vi "WB_print_sub.vi"(1 "최소값":dbl=-2.4903133, 2 "최대값":dbl=1.9686242, 3 "배열":dbl[][](array[numeric])) -> (0 "?":dbl[][](graph)=[[0.019402362, -0.056784116, 0.07198692, 0.023335427, 0.01416415, 0.050220422, -0.07103005, 0.081241615, -0.073664345, -0.05044797, -0.05076698, 0.06311553, 0.061175354, 0.052017786, -0.048248764, -0.08574579, 0.03520029, 0.001996823, 0.04126946, -0.043121457, 0.084707774, -0.06773842, 0.070435666, 0.019763917, -0.059031256, -0.03149846, -0.08095915, 0.004533172], [0.028954692, -0.025707066, -0.05200914, -0.003957868, 0.023727901, -0.06592558, -0.02315136, -0.2734161, -0.20163584, -0.36126682, -0.3774755, -0.14096943, -0.2054312, -0.3512236, 0.33971533, 0.25994176, -0.46906397, -0.70744854, -0.19329818, -0.088722445, 0.036387537, 0.0862372, 0.016047418, 0.06599588, 0.012692414, -0.077935, 0.05922284, 0.05609662], [0.013729125, 0.08213016, 0.06034646, -0.05076416, 0.06025117, -0.15579464, -0.16772258, -0.3223184, -0.37558174, -0.3752564, -0.67335427, -0.49895945, -0.08313592, 0.2052238, 0.2807211, 0.57371145, 0.41389152, -0.17161524, -0.61246336, -0.5017266, -0.50128746, -0.53516656, -0.27541342, -0.3253776, -0.19609226, -0.11948956, -0.012640931, -0.0647767], [-0.015670069, -0.06668488, 0.28268385, 0.20505649, -0.23857276, -0.39677197, -0.38728097, -0.40845335, -0.7503476, -0.4884504, -0.6518539, -0.7594363, -0.24838643, -0.16143909, -0.45154887, -0.02543016, 0.003746802, -0.37966758, -0.49458778, -0.44614837, -0.5836974, -0.41483384, -0.53961504, -0.81955177, -0.83781636, -0.50216895, -0.26348847, -0.076926686], [0.05106411, -0.07743591, 0.26234427, 0.2574695, 0.16226213, -0.46701786, -0.42931813, -0.2339498, -0.14295034, -0.2446104, 0.02086417, -0.32185107, -0.104272395, 0.15050568, 0.027467467, 0.03022217, -0.108522505, -0.27108124, -0.11329941, 0.026872164, 0.048474103, -0.027454505, -0.25504008, -0.26145422, -0.76783425, -0.92602754, -0.58093053, -0.37015644], [0.076194845, -0.034185234, 0.40671673, 0.37028506, 0.41466984, -0.31411722, -0.61910045, -0.59914446, -0.7287402, -0.5391061, -0.2669772, -0.44680798, -0.33798522, -0.1343784, -0.07999179, 0.089457855, -0.19059445, -0.3474572, -0.2032107, -0.083512895, -0.0830359, 0.221656, 0.19037572, 0.12669519, -0.074350126, -1.1324757, -0.4394831, -0.30350068], [-0.032071892, 0.05306862, -0.2989132, 0.21729691, 0.3500755, -0.73872447, -0.8738451, -0.9976445, -0.5223479, -0.3658319, -0.2307682, -0.034148972, -0.13845769, -0.18013148, -0.2361024, -0.31985897, -0.43676993, -0.34739915, -0.06262585, -0.18276054, 0.06466541, 0.08421242, 0.07748312, 0.11180859, -0.21580644, -1.4230266, -0.44195205, -0.3313512], [0.038363524, -0.30228248, -0.21182631, -0.057430062, -0.16909048, -0.92691547, -1.1927773, -0.59489316, -0.5452894, -0.23881502, -0.037728827, -0.038009986, 0.02855738, -0.09971486, -0.14617823, -0.3563637, -0.3384605, -0.24687314, -0.11111135, 0.07221237, 0.033493813, -0.005995454, -0.036368825, -0.15205514, -0.9522951, -1.3690672, -0.43376705, -0.36297065], [0.04789371, -0.27008292, -0.36039582, 0.21856155, -0.37664315, -1.0078262, -0.7442325, -0.44629014, -0.74698794, -0.41905984, -0.084661156, -0.21115676, -0.017576342, 0.072085276, 0.10647539, -0.055365387, -0.1613902, 0.027296007, -0.10239959, -0.034265842, -0.1916164, -0.20936437, -0.24815829, -0.66299695, -1.2413676, -1.1379274, -0.4866338, -0.21672283], [-0.03621333, -0.32016924, -0.35166052, -0.19059004, -0.7421054, -0.6603438, -0.2594525, -0.28854498, -0.54254127, -0.586046, -0.18177606, -0.035845097, -0.14068633, 0.021429166, 0.24718617, 0.54646474, 0.2706092, -0.023800315, -0.11697391, -0.32499748, -0.3964098, -0.17136137, -0.378053, -0.8393874, -1.0225842, -1.1827171, -0.2501431, -0.12847507], [0.045761995, 0.080762595, -0.27182245, -0.26441163, -0.6160039, -0.8418736, -0.5958423, -0.41623044, -0.29561433, -0.5286718, -0.13444705, -0.048691455, -0.06864151, 0.1826969, 0.6635885, 0.802045, 0.32688302, 0.0874516, -0.17387727, -0.2563993, -0.30054188, -0.096157655, -0.508509, -0.99769956, -1.4066856, -0.29529485, -0.37173674, 0.21905021], [-0.07151403, 0.28909746, 0.38781136, -0.26616985, -0.4273282, -0.41229233, -0.8697481, -0.5518835, -0.31008196, -0.2774829, -0.26617262, -0.15640731, -0.10818419, 0.24041, 0.79541355, 0.70669216, 0.28055012, -0.16330147, -0.10160323, -0.2256082, -0.35910672, -0.39827135, -0.650711, -0.62799734, -0.90181077, -0.107671015, -0.36124784, 0.22384478], [0.078392126, 0.031860493, -0.25298005, 0.095670424, -0.14538823, -0.16609928, -0.31244653, -0.12862818, -0.22139308, 0.07183458, -0.32371405, -0.4855172, -0.08327049, 0.3265337, 0.78024745, 0.60129076, 0.18782617, -0.01853502, -0.07388906, -0.40313932, -0.40507895, -0.009898128, -0.27054566, -0.34444198, -0.7273675, -0.2863849, -0.42149025, 0.041592613], [0.21364997, -0.007809334, -0.15489164, 0.41396883, 0.031446937, -0.14940584, -0.2472778, -0.22871476, 0.32454446, -0.028100867, -0.65081227, -0.552141, -0.016222754, 0.30621958, 0.6353163, 0.6064552, 0.1867488, 0.19777592, -0.1788572, -0.6515122, -0.52407956, -0.11200111, -0.4531192, -0.592242, -0.7931037, -0.4800189, -0.43356013, -0.09559373], [0.041847475, 0.020147942, 0.28636876, 0.3035632, 0.3176007, -0.2528747, -0.78754634, -0.18334779, 0.092457, -0.2796707, -0.74587876, -0.5658111, 0.000195621, 0.30102542, 0.6712702, 0.49273783, 0.22195052, -0.16626519, -0.41114998, -0.5848261, -0.4108646, -0.18204437, -0.21483289, -0.14545862, 0.025073398, -0.07972018, 0.14786825, 0.0397756], [0.007859804, 0.004111923, 0.3043381, 0.38932654, 0.4320326, -0.4698006, -0.9373428, -0.04405305, -0.023937216, -0.47727737, -0.483351, -0.083477095, 0.21139918, 0.5714958, 0.8108114, 0.20742717, 0.18971094, -0.5720092, -0.8250202, -1.2184142, -1.1274087, -0.2133971, -0.31071362, -0.5049326, -0.18142083, -0.24756274, 0.030007659, -0.2307325], [0.034503534, 0.30741704, 0.3961975, -0.028361622, 0.16783519, -0.7315894, -0.8071333, -0.37223402, -0.27927428, 0.0536947, -0.21464181, -0.053445697, -0.011839257, 0.4265288, 0.6584135, 0.006877806, -0.117410704, -0.88479674, -0.9323623, -1.306204, -0.35932663, -0.20176698, -0.26285505, -0.79386646, -0.49305102, -0.92046, -0.20253757, -0.4379618], [0.0269147, 0.26754153, 0.17135796, -0.20873298, 0.11994213, -0.8284057, -0.88438743, -0.502535, -0.112462565, -0.18551545, -0.047672696, -0.33874467, 0.074904464, 0.40984982, 0.6418728, -0.05189987, -0.48060784, -0.8236671, -0.42577484, -0.22257994, -0.042787, -0.009383095, 0.05736418, -0.19098903, -0.4478566, -1.0353278, -0.020705368, -0.39874083], [0.1397072, 0.45009655, -0.064224996, -0.3019297, -0.8661276, -1.3250548, -1.2598255, -0.5243417, -0.058559388, -0.09852703, -0.3158096, -0.19829708, -0.0714448, 0.22167754, 0.2854061, -0.3002683, -0.59488386, -0.2821777, 0.028929045, 0.05826009, 0.33111486, 0.16548227, -0.21062346, -0.25565898, -0.5472606, -0.28622505, 0.18191522, 0.41757488], [0.23692198, 0.29008064, 0.082759045, -0.002741147, -0.8795839, -1.4149228, -0.5514523, -0.000486821, -0.03483119, 0.06705211, -0.12580939, -0.05553379, 0.0186108, 0.24032596, 0.005597983, -0.06941267, 0.16518432, -0.06645737, 0.19766212, 0.38022786, 0.09240109, -0.013227117, -0.25650293, -0.044998907, 0.12227106, 0.17152156, 0.18103345, 0.41024154], [-0.06607313, -0.020586662, -0.3017442, -0.48487973, -0.623512, -0.7337084, -0.13421166, -0.012992498, 0.19180049, 0.10447126, 0.17092228, 0.22486123, 0.0976739, -0.06349748, 0.106518574, 0.05040216, 0.36003187, 0.276737, 0.49036795, 0.30218476, 0.11204288, 0.12559855, -0.35291293, -0.35144538, 0.014885792, 0.005825452, 0.29019934, 0.21266916], [0.27878812, 0.15665133, -0.003313494, 0.12400361, 0.2629784, 0.37134543, 0.2215543, 0.11155561, 0.15902479, 0.20833528, 0.32967663, 0.037060052, -0.08899602, -0.16459641, 0.1264346, 0.2089554, 0.1434192, 0.06803246, 0.4307756, 0.24303465, 0.18769139, 0.25835752, -0.4969824, -0.73953736, -0.10242521, -0.112113826, 0.003337876, -0.0351161], [0.28544542, 0.1967097, -0.006959932, -0.20673351, 0.026372466, 0.94482493, 0.4533628, 0.026862903, 0.17517203, 0.20571615, -0.039798018, -0.29742217, -0.3459068, -0.36140463, 0.0369192, -0.012902046, 0.048173387, 0.33128628, 0.47379583, 0.3349553, 0.25610295, -0.08089572, -0.5139698, -0.07225746, -0.5919201, 0.19126964, 0.36402228, 0.075980864], [-0.04799637, 0.022139437, -0.08066415, -0.45350027, -0.36171135, 0.48501188, 0.40540573, 0.07247676, -0.002596119, -0.068791166, -0.120647185, -0.13058528, 0.06652875, -0.15032628, -0.2481706, 0.10068886, 0.17316899, 0.44682083, 0.07280411, 0.03211489, -0.29994527, -0.5088104, -0.42009258, -0.87431175, -0.06847369, 0.17766212, 0.52052814, 0.008205421], [-0.08633989, 0.050158076, -0.10934232, -0.43204042, -0.7932491, -0.085638694, -0.04620965, -0.21960713, -0.3608294, -0.15517698, -0.31756258, -0.34403557, -0.22502212, -0.47006503, -0.24211344, -0.36654466, -0.69102883, -0.022553908, -0.07223295, 0.08607136, -0.40333796, -0.29468244, -0.44569877, -0.06304068, -0.17344941, 0.35010365, 0.27814704, 0.006576605], [-0.05087135, -0.08338762, -0.030791346, -0.4005939, -0.85698, -0.90138805, -0.79291576, -0.93168545, -0.4134845, -0.50070626, -1.4878545, -1.4652365, -0.84761375, -0.87468684, -0.76639235, -1.0541568, -1.6761183, -1.4510397, -1.2478479, -1.2098646, -0.7164307, -0.44639748, -0.21093823, -0.2979916, -0.3668138, 0.048997097, -0.07975093, -0.07314849], [0.064261444, -0.012364283, 0.051179014, -0.1375661, -0.27762103, -0.35109448, -0.44071844, -0.44467148, -0.74206126, -0.91204447, -0.8158255, -0.9406752, -1.1595905, -0.9655593, -1.0871019, -0.8791337, -0.9534564, -0.90534633, -0.59114176, -0.49164557, -0.23583324, -0.3829994, -0.38570908, -0.29194045, -0.00429406, -0.012259826, 0.02296777, -0.039393578], [-0.041495476, -0.061708644, 0.040426068, -0.068808526, -0.008004427, -0.0743755, -0.03914054, -0.000495799, -0.004151344, -0.068212785, -0.31595376, -0.40251288, -0.2163812, -0.30054742, -0.363434, -0.025332911, -0.055431835, -0.33812305, -0.25177604, -0.26286864, 0.004775614, -0.01410728, -0.011602685, 0.067894004, -0.042782366, -0.043303426, 0.050262995, -0.00822515], [0.0, 0.0, 0.0, 0.0, 0.0, 0.0, 0.0, 0.0, 0.0, 0.0, 0.0, 0.0, 0.0, 0.0, 0.0, 0.0, 0.0, 0.0, 0.0, 0.0, 0.0, 0.0, 0.0, 0.0, 0.0, 0.0, 0.0, 0.6847913]])   [LabVIEW 2021]
panel:
  out "범위":dbl[](array[numeric])=[-2.4903133, 0.0, 2.4903133]
  in  "색선택":u32[](array[colorbox])=[16711680, 0, 65280]
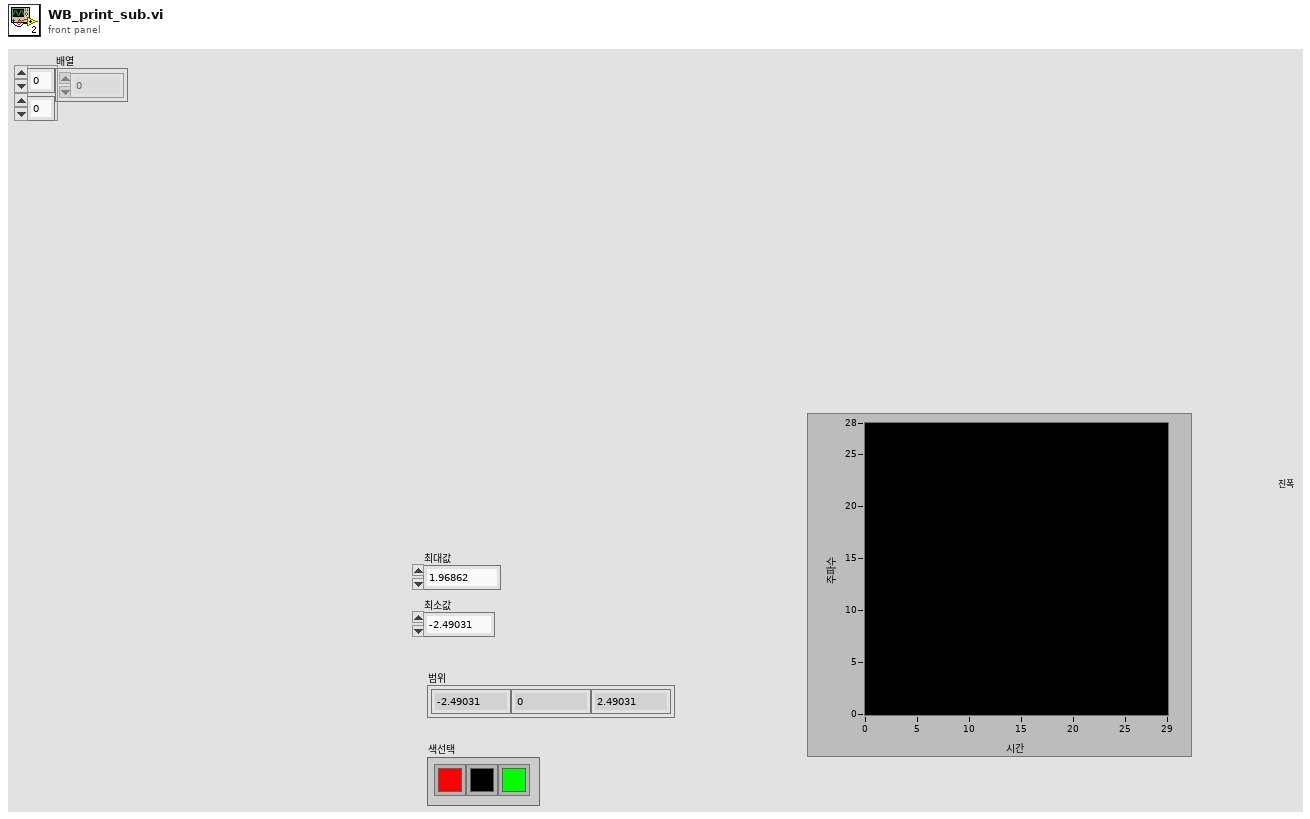
[diagram p1: front panel]
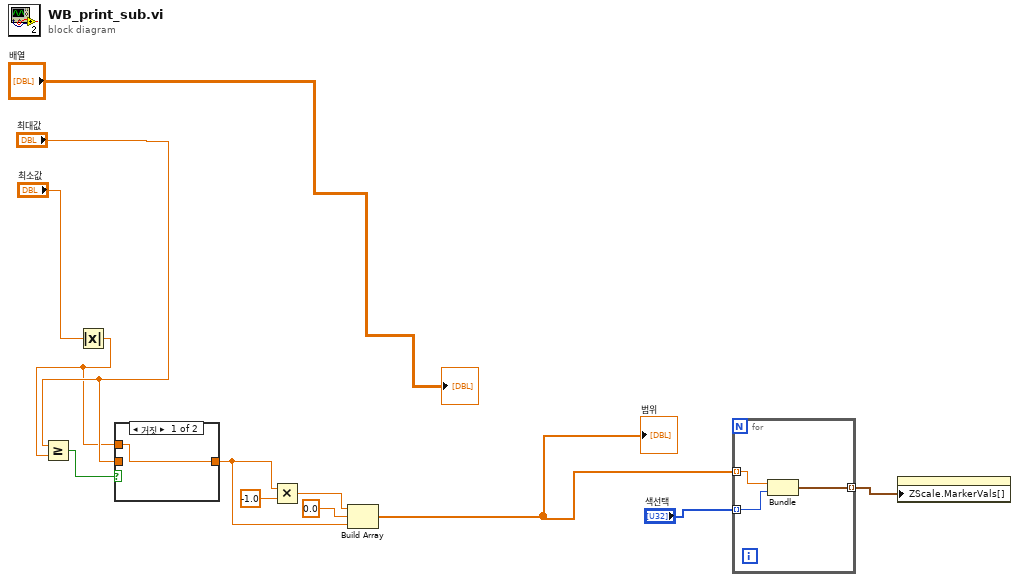
[diagram p0: block diagram]
diagram:
  n1 = Absolute Value(x="최소값") -> (abs(x)=w5:dbl)
  n2 = Greater Or Equal?(x="최대값", y=w5) -> (x >= y?=w10:bool)
  n3 = case shown="거짓" w10 {
    tunnel: "최대값" -> [_ w14]
    tunnel: [w13 w14] -> w6
    tunnel: w5 -> [w13 _]
    frame False {
    }
    frame True {
    }
  }
  n4 = Multiply(x=w6, y=-1.0) -> (x*y=w7:dbl)
  n5 = Build Array(w7, 0.0 ("원소"), w6) -> (w3:dbl[])
  "범위" <- w3
  n6 = for {
    tunnel: w3 -> [w17] mode=indexing
    tunnel: "색선택" -> [w16] mode=indexing
    tunnel: [w15] -> w1 mode=indexing
    n7 = Bundle("최대값"=w17, "색 상자"=w16) -> (w15:cluster{"최대값":dbl, "색 상자":u32})  [unwired: 1 in]
  }
  n8 = property class="IntGraph (엄격한)"("ZScale.MarkerVals[]"=w1) -> ()  [unwired: 2 in, 2 out]
  "?" <- "배열"
